vi "uA_daq_Re_Init_daq_follow_input.vi"(8 "error in (no error)":errorcluster, 9 "Acquire Mode":enum16{"Streaming", "Read All", "Stop"}(ring), 10 "USB":tag, 11 "Range_shunt":T1) -> (0 "error out":errorcluster, 3 "Refnum out":refnum<k21>)   [LabVIEW 2015]
uses:
  Range_Shunt_selector.ctl
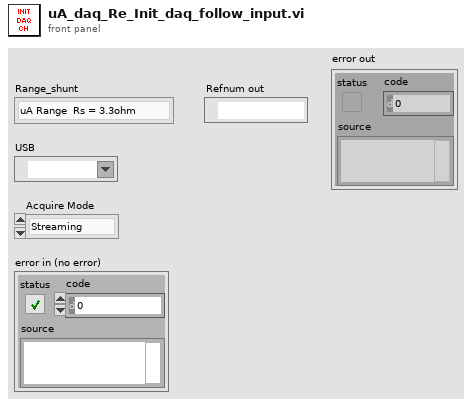
[diagram p1: front panel]
types:
  T1 = typedef "Range_Shunt_selector.ctl" = enum16{"uA Range  Rs = 3.3ohm", "mA Range Rs = 3.3Ohm", "mA Range Rs = 1Ohm", "mA Range Rs = 1Ohm - X2"}
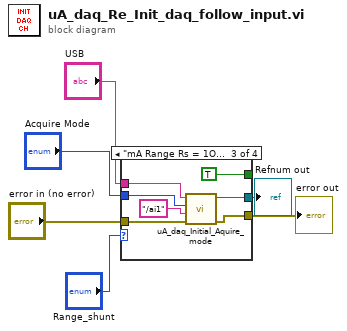
[diagram p0: block diagram]
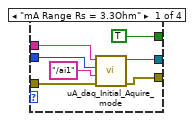
[diagram p2: hidden frame]
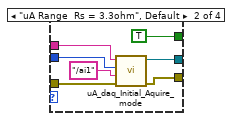
[diagram p3: hidden frame]
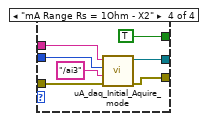
[diagram p4: hidden frame]
diagram:
  n1 = case shown="\"mA Range Rs = 1Ohm\"" "Range_shunt" {
    tunnel: [w13 w20 w27 w34] -> w3
    tunnel: [TRUE TRUE TRUE TRUE] -> _
    tunnel: "Acquire Mode" -> [w9 w16 w23 w31]
    tunnel: "error in (no error)" -> [w8 w15 w22 w30]
    tunnel: "USB" -> [w10 w17 w24 w29]
    tunnel: [w7 w14 w21 w28] -> w1
    frame "mA Range Rs = 3.3Ohm" {
      n2 = call "uA_daq_Initial_Aquire_mode.vi"("error in"=w8, "ADC_Ch"="/ai1", "Acquire Mode"=w9, "USB DAQ"=w10) -> ("error out"=w7:errorcluster, "Refnum out"=w13:refnum<k21>)  [unwired: 6 in]
    }
    frame "uA Range  Rs = 3.3ohm", Default {
      n3 = call "uA_daq_Initial_Aquire_mode.vi"("error in"=w15, "ADC_Ch"="/ai1", "Acquire Mode"=w16, "USB DAQ"=w17) -> ("error out"=w14:errorcluster, "Refnum out"=w20:refnum<k21>)  [unwired: 6 in]
    }
    frame "mA Range Rs = 1Ohm" {
      n4 = call "uA_daq_Initial_Aquire_mode.vi"("error in"=w22, "ADC_Ch"="/ai1", "Acquire Mode"=w23, "USB DAQ"=w24) -> ("error out"=w21:errorcluster, "Refnum out"=w27:refnum<k21>)  [unwired: 6 in]
    }
    frame "mA Range Rs = 1Ohm - X2" {
      n5 = call "uA_daq_Initial_Aquire_mode.vi"("error in"=w30, "ADC_Ch"="/ai3", "Acquire Mode"=w31, "USB DAQ"=w29) -> ("error out"=w28:errorcluster, "Refnum out"=w34:refnum<k21>)  [unwired: 6 in]
    }
  }
  "Refnum out" <- w3
  "error out" <- w1
